vi "OpenSubpanelHandler.vi"(8 "error in (no error)":errorcluster, 10 "GUID":string, 11 "SMO.UI.MAUI in":refnum<class "MAUI.lvclass">) -> (0 "error out":errorcluster, 3 "SMO.UI.MAUI out":refnum<class "MAUI.lvclass">)   [LabVIEW 2019, in "MAUI.lvclass"]
uses:
  MAUI.lvclass
  MAUI.lvclass/MAUI.ctl
  <userlib>/LevyLab/Embedded UI/SMO.UI.Embedded/Embedded UI.lvclass
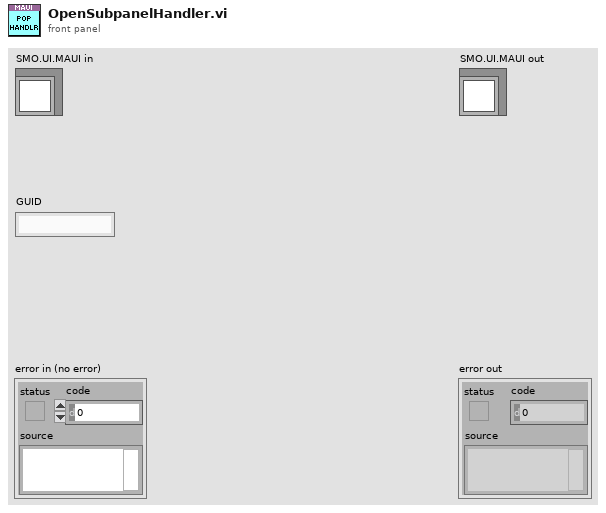
[diagram p1: front panel]
types:
  T1 = typedef "MAUI.lvclass/PanelData.ctl" = cluster{"SubPanel":refnum<vi>, "Ring":refnum<vi>, "Active":i32}
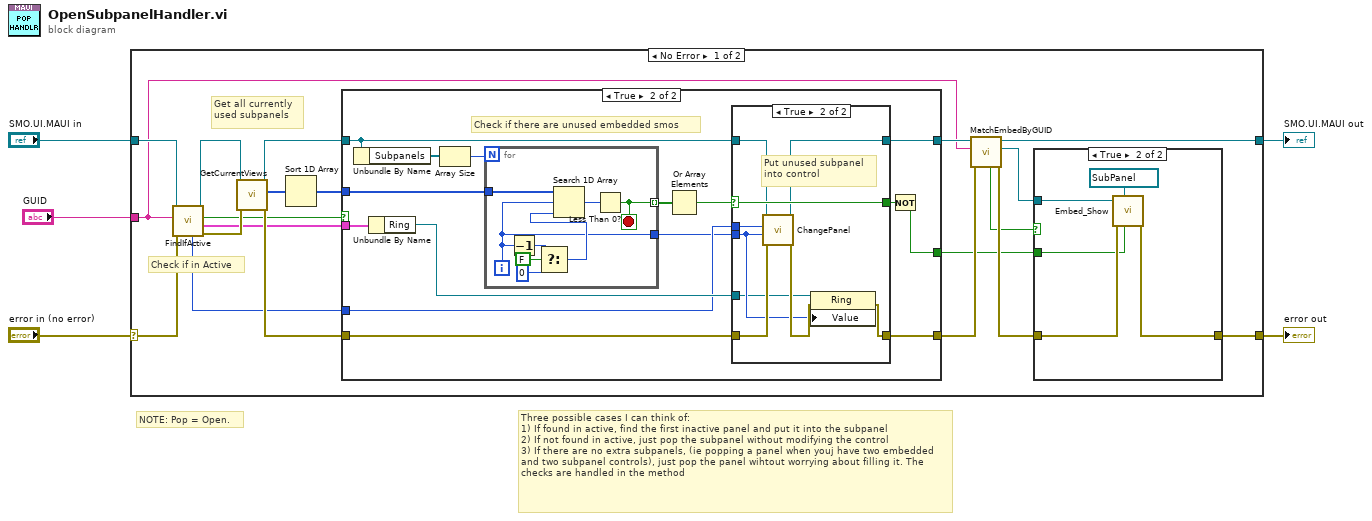
[diagram p0: block diagram]
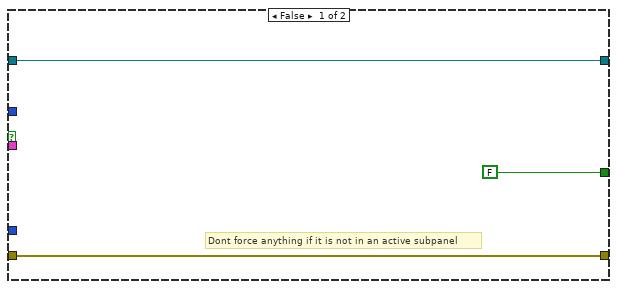
[diagram p3: hidden frame]
diagram:
  # "NOTE: Pop = Open."
  # "Three possible cases I can think of:\n1) If found in active, find the first inactive panel and put it into the subpanel\n2) If not found in active, just pop the subpanel without modifying the control\n3) If there are no extra subpanels, (ie popping a panel when youj have two embedded and two subpanel controls), just pop the panel wihtout worrying about filling it. The checks are handled in the method"
  n1 = case shown="No Error" "error in (no error)" {
    selector: "error in (no error)" -> [w25 w71]
    tunnel: [w20 w71] -> w4
    tunnel: [w10 w70] -> w2
    tunnel: "SMO.UI.MAUI in" -> [w19 w70]
    tunnel: "GUID" -> [w6 _]
    frame No Error {
      # "Get all currently used subpanels"
      # "Check if in Active"
      n2 = call "FindIfActive.vi"("error in (no error)"=w25, "GUID"=w6, "SMO.UI.MAUI in"=w19) -> ("error out"=w23:errorcluster, "Panel"=w14:T1, "Found?"=w15:bool, "SMO.UI.MAUI out"=w18:refnum<class "MAUI.lvclass">, "Panel Index"=w12:i32)  [unwired: 4 in]
      n3 = call "GetCurrentViews.vi"("error in (no error)"=w23, "SMO.UI.MAUI in"=w18) -> ("error out"=w24:errorcluster, "Current Views"=w17:i32[], "SMO.UI.MAUI out"=w16:refnum<class "MAUI.lvclass">)  [unwired: 7 in]
      n4 = Sort 1D Array(array=w17) -> (sorted array=w13:i32[])
      n5 = case shown="True" w15 {
        tunnel: w16 -> [w33 w46]
        tunnel: [w33 w47] -> w11
        tunnel: w14 -> [_ w42]
        tunnel: w13 -> [_ w45]
        tunnel: w12 -> [_ w40]
        tunnel: w24 -> [w34 w49]
        tunnel: [w34 w48] -> w22
        tunnel: [FALSE w37] -> w7
        frame False {
          # "Dont force anything if it is not in an active subpanel"
        }
        frame True {
          # "Check if there are unused embedded smos"
          n6 = Unbundle By Name(w46) -> ("Subpanels"=w36:refnum<class "Embedded UI.lvclass">[])
          n7 = Unbundle By Name(w42) -> ("Ring"=w41:refnum<vi>)
          n8 = Array Size(array=w36) -> (size(s)=w35:i32)
          n9 = for {
            N: w35 -> [_]
            tunnel: w45 -> [w57]
            tunnel: [w55] -> w44 mode=indexing
            tunnel: [w50] -> w39
            i -> [w50]
            stop <- w55 stop-if-true
            n10 = Decrement(x=w50) -> (x-1=w54:i32)
            n11 = Select(t=w54, s=FALSE, f=0) -> (s? t:f=w51:i32)
            n12 = Search 1D Array(1D array=w57, element=w50, start index (0)=w51) -> (index of element=w56:i32)
            n13 = Less Than 0?(x=w56) -> (x < 0?=w55:bool)
          }
          n14 = Or Array Elements(Boolean array=w44) -> (logical OR=w43:bool)
          n15 = case shown="True" w43 {
            selector: w43 -> [w58 w66]
            tunnel: w46 -> [w59 w64]
            tunnel: [w59 w65] -> w47
            tunnel: w41 -> [_ w61]
            tunnel: w40 -> [_ w63]
            tunnel: w39 -> [_ w62]
            tunnel: [w58 w66] -> w38
            tunnel: w49 -> [w60 w69]
            tunnel: [w60 w68] -> w48
            frame False {
            }
            frame True {
              # "Put unused subpanel\ninto control"
              n16 = call "ChangePanel.vi"("error in (no error)"=w69, "New Active Index"=w62, "Panel Index"=w63, "MAUI in"=w64) -> ("error out"=w67:errorcluster, "MAUI out"=w65:refnum<class "MAUI.lvclass">)  [unwired: 6 in]
              n17 = property on="Property Node" class="Ring"(reference=w61, error in=w67, "Value"=w62) -> (error out=w68:errorcluster)  [unwired: 1 out]
            }
          }
          n18 = Not(x=w38) -> (.not. x?=w37:bool)
        }
      }
      n19 = call "MatchEmbedByGUID.vi"("error in (no error)"=w22, "GUID"=w6, "SMO.UI.MAUI in"=w11) -> ("error out"=w21:errorcluster, "Value"=w8:refnum<class "Embedded UI.lvclass">, "SMO.UI.MAUI out"=w10:refnum<class "MAUI.lvclass">, "Found?"=w9:bool)  [unwired: 4 in, 1 out]
      n20 = case shown="True" w9 {
        tunnel: w21 -> [w26 w30]
        tunnel: [w26 w31] -> w20
        tunnel: w8 -> [_ w29]
        tunnel: w7 -> [_ w27]
        frame False {
          # "If you dont find subpanel,\nDont stick it into reference."
        }
        frame True {
          n21 = call <userlib>:"Embed_Show.vi"("Force?"=w27, "Sub Panel"=refnum<vi> refnum, "error in (no error)"=w30, "EmbeddedSMO in"=w29) -> ("error out"=w31:errorcluster)  [unwired: 6 in, 1 out]
        }
      }
    }
    frame Error {
    }
  }
  "error out" <- w4
  "SMO.UI.MAUI out" <- w2
